vi "Stable Demonstator.vi"() -> ()   [LabVIEW 2011]
panel:
  out "Monitor":cluster{i16, i16}(graph)
  in  "Signal Input":bool
  out "Stable":bool
  in  "Eval Period (sec)":dbl(knob)=0.5044674819294696 scale=0.0..1.0
  # "This will check if a Boolean stays 'on' for a settable pulse width,\nand outputs a 'Stable' Boolean when this condition is met"
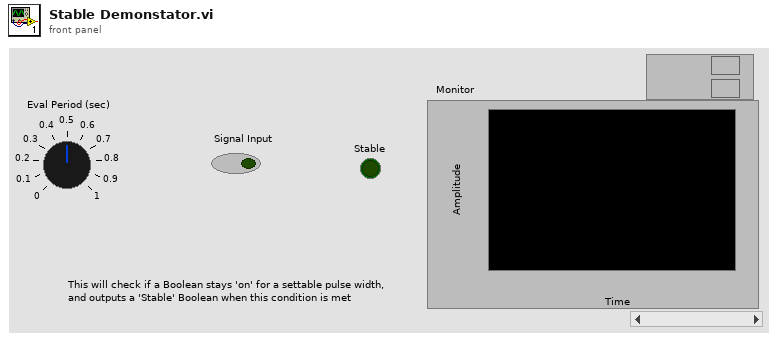
[diagram p1: front panel]
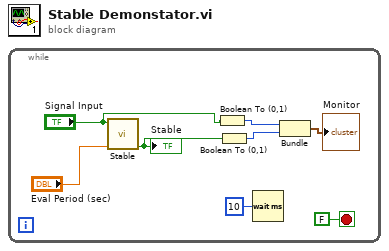
[diagram p0: block diagram]
diagram:
  n1 = while {
    stop <- FALSE stop-if-true
    n2 = call "Stable.vi"("Eval Period (sec)"="Eval Period (sec)", "Signal Input"="Signal Input") -> ("Stable"=w1:bool)  [unwired: 9 in]
    "Stable" <- w1
    n3 = Boolean To (0,1)(Boolean="Signal Input") -> (0, 1=w3:i16)
    n4 = Boolean To (0,1)(Boolean=w1) -> (0, 1=w4:i16)
    n5 = Wait (ms)(milliseconds to wait=u32 10) -> ()  [unwired: 1 out]
    n6 = Bundle(w3, w4) -> (→"Monitor":cluster{i16, i16})  [unwired: 1 out]
  }
